vi "Create Calendar Folder Tree.vi"(7 "Start Time Stamp":timestamp, 8 "Error In":errorcluster, 11 "Base Log Folder":path) -> (0 "Error Out":errorcluster, 3 "Calendar Folder Tree":path)   [LabVIEW 2017, in "Logger.lvlib" / "File.lvlib"]
uses:
  File.lvlib
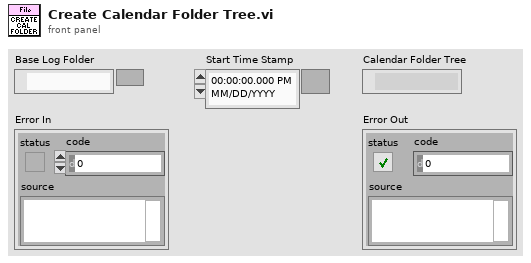
[diagram p1: front panel]
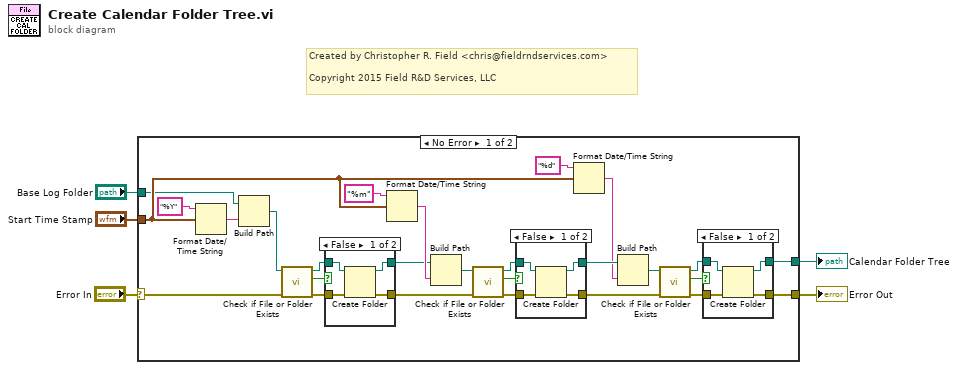
[diagram p0: block diagram]
diagram:
  # "Created by Christopher R. Field <chris@fieldrndservices.com>\n\nCopyright 2015 Field R&D Services, LLC"
  n1 = case shown="No Error" "Error In" {
    selector: "Error In" -> [w25 w51]
    tunnel: "Start Time Stamp" -> [w28 _]
    tunnel: "Base Log Folder" -> [w27 w52]
    tunnel: [w7 w52] -> w2
    tunnel: [w6 w51] -> w1
    frame No Error {
      n2 = Format Date/Time String(time format string (%c)="%Y", seconds (now)=w28) -> (date/time string=w31:string)  [unwired: 1 in]
      n3 = Build Path(base path=w27, name or relative path=w31) -> (appended path=w26:path)
      n4 = call <vilib>:"Check if File or Folder Exists.vi"("error in (no error)"=w25, "path"=w26) -> ("error out"=w22:errorcluster, "file or folder exists?"=w24:bool, "dup path"=w23:path)  [unwired: 7 in]
      n5 = case shown="False" w24 {
        tunnel: w23 -> [w48 w50]
        tunnel: w22 -> [w47 w49]
        tunnel: [w46 w50] -> w20
        tunnel: [w45 w49] -> w12
        frame False {
          n6 = Create Folder(path (use dialog)=w48, error in=w47) -> (created path=w46:path, error out=w45:errorcluster)  [unwired: 1 in, 1 out]
        }
        frame True {
        }
      }
      n7 = Format Date/Time String(time format string (%c)="%m", seconds (now)=w28) -> (date/time string=w21:string)  [unwired: 1 in]
      n8 = Build Path(base path=w20, name or relative path=w21) -> (appended path=w13:path)
      n9 = call <vilib>:"Check if File or Folder Exists.vi"("error in (no error)"=w12, "path"=w13) -> ("error out"=w17:errorcluster, "file or folder exists?"=w19:bool, "dup path"=w18:path)  [unwired: 7 in]
      n10 = case shown="False" w19 {
        tunnel: w18 -> [w42 w44]
        tunnel: w17 -> [w41 w43]
        tunnel: [w40 w44] -> w11
        tunnel: [w39 w43] -> w8
        frame False {
          n11 = Create Folder(path (use dialog)=w42, error in=w41) -> (created path=w40:path, error out=w39:errorcluster)  [unwired: 1 in, 1 out]
        }
        frame True {
        }
      }
      n12 = Format Date/Time String(time format string (%c)="%d", seconds (now)=w28) -> (date/time string=w10:string)  [unwired: 1 in]
      n13 = Build Path(base path=w11, name or relative path=w10) -> (appended path=w9:path)
      n14 = call <vilib>:"Check if File or Folder Exists.vi"("error in (no error)"=w8, "path"=w9) -> ("error out"=w14:errorcluster, "file or folder exists?"=w16:bool, "dup path"=w15:path)  [unwired: 7 in]
      n15 = case shown="False" w16 {
        tunnel: w15 -> [w36 w38]
        tunnel: w14 -> [w35 w37]
        tunnel: [w34 w38] -> w7
        tunnel: [w33 w37] -> w6
        frame False {
          n16 = Create Folder(path (use dialog)=w36, error in=w35) -> (created path=w34:path, error out=w33:errorcluster)  [unwired: 1 in, 1 out]
        }
        frame True {
        }
      }
    }
    frame Error {
    }
  }
  "Calendar Folder Tree" <- w2
  "Error Out" <- w1
